vi "Agilent DMM Read Measurement Type.vi"(8 "error in (no error)":errorcluster, 11 "VISA Resource Name":refnum<visa-resource-name>) -> (0 "error out":errorcluster, 2 "Measurement Type":T1, 3 "dup VISA Resource Name":refnum<visa-resource-name>)   [LabVIEW 2011]
doc: "This VI for the HP 8753 is used to read the sweep type.\n\n0 LINEAR FREQ\n1 LOG FREQ\n2 LIST FREQ\n3 CW TIME\n4 POWER SWEEP"
uses:
  TypeDefs/Agilent DMM Measurement Type.ctl
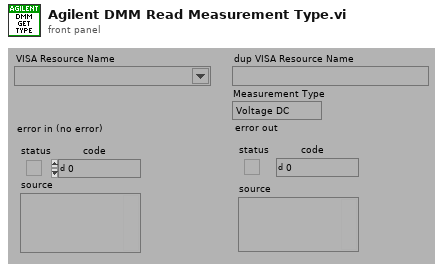
[diagram p1: front panel]
types:
  T1 = typedef "Agilent DMM Measurement Type.ctl" = enum16{"Voltage DC", "Voltage DC Ratio", "Voltage AC", "Current DC", "Current AC", "Resistance", "Fresistance", "Frequency", "Period", "Continuity", "Diode"}
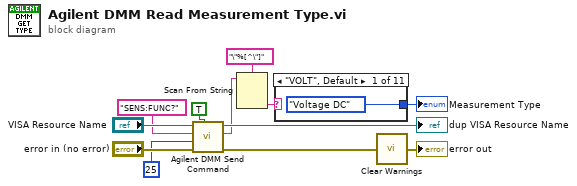
[diagram p0: block diagram]
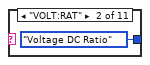
[diagram p2: hidden frame]
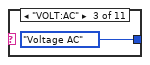
[diagram p3: hidden frame]
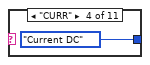
[diagram p4: hidden frame]
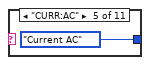
[diagram p5: hidden frame]
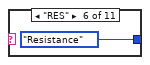
[diagram p6: hidden frame]
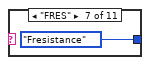
[diagram p7: hidden frame]
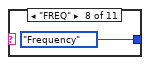
[diagram p8: hidden frame]
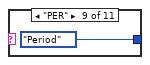
[diagram p9: hidden frame]
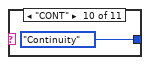
[diagram p10: hidden frame]
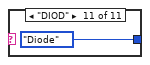
[diagram p11: hidden frame]
diagram:
  n1 = call "Agilent DMM Send Command.vi"("Read? (F)"=TRUE, "error in (no error)"="error in (no error)", "Byte Count"=u32 25, "Command"="SENS:FUNC?" ("write buffer"), "VISA Resource Name"="VISA Resource Name") -> ("error out"=w3:errorcluster, "Data Read"=w4:string, "dup VISA Resource Name"=→"dup VISA Resource Name":refnum<visa-resource-name>)  [unwired: 4 out]
  n2 = Scan From String(format string="\"%[^\"]", input string=w4) -> (output 1=w8:string)  [unwired: 2 in, 4 out]
  n3 = case shown="\"VOLT\", Default" w8 {
    tunnel: [Agilent_DMM_Measurement_Type."Voltage DC" ("Measurement Type") Agilent_DMM_Measurement_Type."Voltage DC Ratio" ("Measurement Type") Agilent_DMM_Measurement_Type."Voltage AC" ("Measurement Type") Agilent_DMM_Measurement_Type."Current DC" ("Measurement Type") Agilent_DMM_Measurement_Type."Current AC" ("Measurement Type") Agilent_DMM_Measurement_Type."Resistance" ("Measurement Type") Agilent_DMM_Measurement_Type."Fresistance" ("Measurement Type") Agilent_DMM_Measurement_Type."Frequency" ("Measurement Type") Agilent_DMM_Measurement_Type."Period" ("Measurement Type") Agilent_DMM_Measurement_Type."Continuity" ("Measurement Type") Agilent_DMM_Measurement_Type."Diode" ("Measurement Type")] -> w9
    frame "VOLT", Default {
    }
    frame "VOLT:RAT" {
    }
    frame "VOLT:AC" {
    }
    frame "CURR" {
    }
    frame "CURR:AC" {
    }
    frame "RES" {
    }
    frame "FRES" {
    }
    frame "FREQ" {
    }
    frame "PER" {
    }
    frame "CONT" {
    }
    frame "DIOD" {
    }
  }
  "Measurement Type" <- w9
  n4 = call "Clear Warnings.vi"("error in (no error)"=w3) -> ("error out"=→"error out":errorcluster)
